vi "Macro Init.vi"(8 "error in (no error)":errorcluster, 10 "Repository Path":path, 11 "Git in":refnum<class "Git.lvclass">) -> (0 "error out":errorcluster, 3 "Git out":refnum<class "Git.lvclass">)   [LabVIEW 2019, in "Git.lvclass"]
uses:
  Git.lvclass
  <vilib>/Hampel Software Engineering/Git API/Git API/GIT-api.lvclass/GIT-api.ctl
  Git.lvclass/Git.ctl
  <vilib>/Hampel Software Engineering/Git API/Git API/GIT-api.lvclass
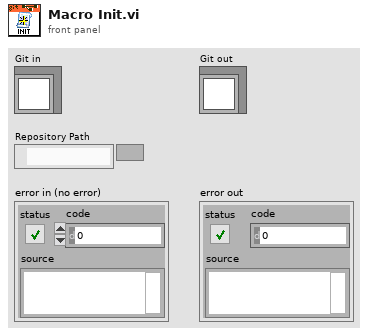
[diagram p1: front panel]
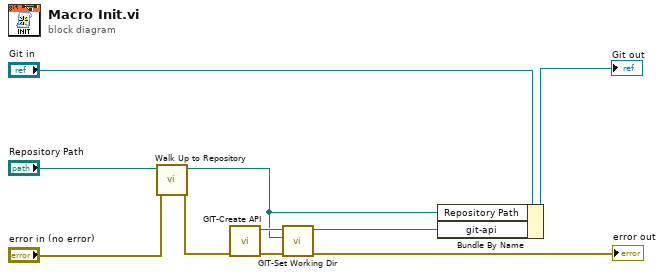
[diagram p0: block diagram]
diagram:
  n1 = call "Walk Up to Repository.vi"("error in (no error)"="error in (no error)", "Build Path"="Repository Path") -> ("error out"=w4:errorcluster, "Repository Path"=w3:path)  [unwired: 8 in]
  n2 = call <vilib>:"GIT-Create API.vi"("error in"=w4) -> ("error out"=w7:errorcluster, "git-api out"=w6:refnum<class "GIT-api.lvclass">)  [unwired: 9 in]
  n3 = call <vilib>:"GIT-Set Working Dir.vi"("error in"=w7, "Working Directory"=w3, "git-api in"=w6) -> ("error out"=→"error out":errorcluster, "git-api out"=w8:refnum<class "GIT-api.lvclass">)  [unwired: 7 in]
  n4 = Bundle By Name(cluster="Git in", "Repository Path"=w3, "git-api"=w8) -> (→"Git out":refnum<class "Git.lvclass">)
